vi "Visualize.vi"() -> ()   [LabVIEW 2018, in "Visualization.lvlib" / "VisualizeAcPwr.lvclass"]
uses:
  VisualizeAcPwr.lvclass
  VisualizeDigitizer/VisualizeDigitizer.lvclass
  VisualizeBase/VisualizeBase_class/Requests/clUserEventType.ctl
  <vilib>/event_ctls.llb/usereventprio.ctl
  <vilib>/Utility/error.llb/Error Cluster From Error Code.vi
  <vilib>/ErrorRing/Error Ring.xnode
  VisualizeBase/VisualizeBase_class/VisualizeBase.lvclass
  <userlib>/NIST/NISTErrorLib/NISTErrorLib.lvlib
  AcPwr/AcPwrModule/AcPwrModule.lvlib
panel:
  in  "Tab Control":enum32{"AC Instruments", "DC Instruments"}(tab)
  out "PacificPower":waveform(dbl)[](graph) caption="4140002"
  out "Chroma AC":waveform(dbl)[](graph) caption="4140003"
  out "NHRDC":waveform(sgl)[](graph) caption="-1"
  out "Chroma DC":waveform(dbl)[](graph) caption="4140003"
  out "ErrorArray":errorcluster[](array[cluster])
  in  "QueuName":string="AcPwrVisQue"
  in  "btnStop":bool
  in  "btnReset":bool
  in  "btnClear":bool
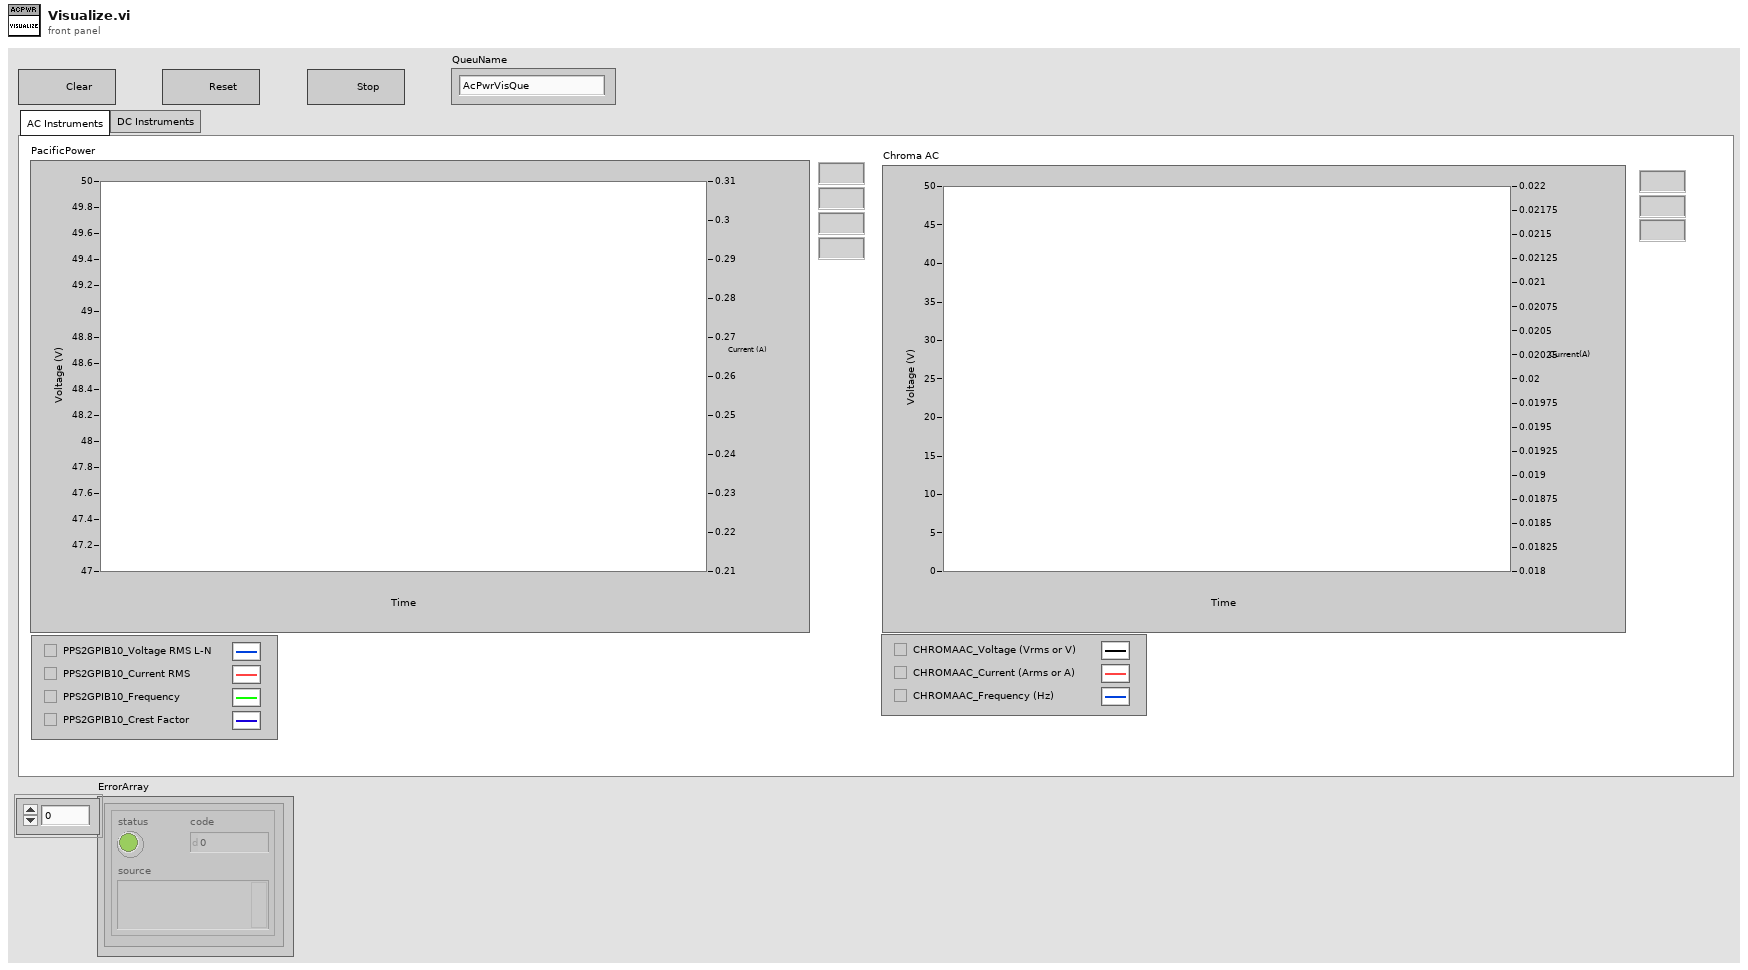
[diagram p1: front panel]
types:
  T1 = typedef "Visualization.lvlib/VisualizeBase.lvclass/clRequestEvents.ctl" = cluster{"StopRequest":refnum<user-event>, "ResetRequest":refnum<user-event>}
  T2 = typedef "AcPwrModule.lvlib/clBroadcastEvents.ctl" = cluster{"DidInit":refnum<user-event>, "StatusUpdate":refnum<user-event>, "ErrorReport":refnum<user-event>, "DidStop":refnum<user-event>, "PathToINI":refnum<user-event>, "Measurements":refnum<user-event>, "LoadConfigFile":refnum<user-event>}
  T3 = typedef "Visualization.lvlib/VisualizeBase.lvclass/clUserEventType.ctl" = cluster{"BusIndex":i8, "Data":variant}
  T4 = typedef "usereventprio.ctl" = enum32{"high priority", "normal priority"}
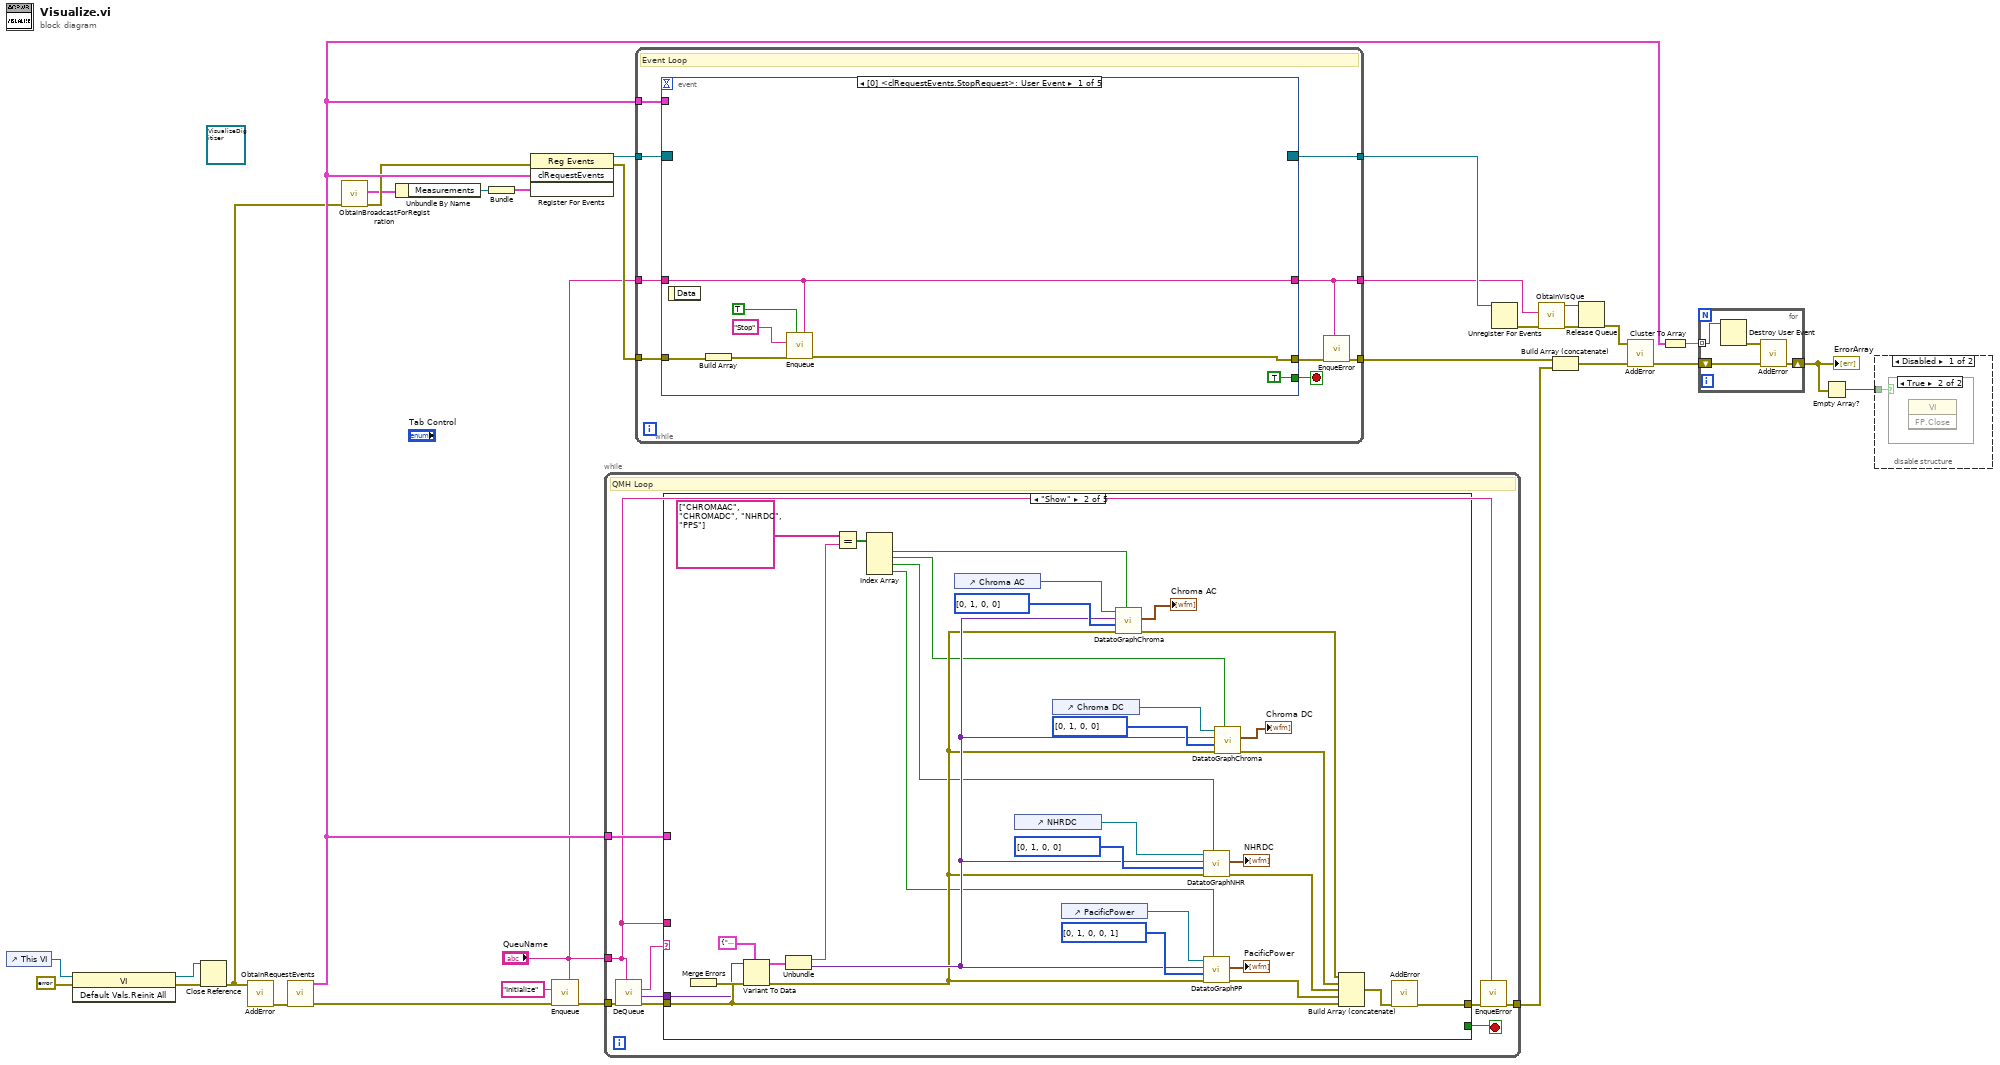
[diagram p0: block diagram]
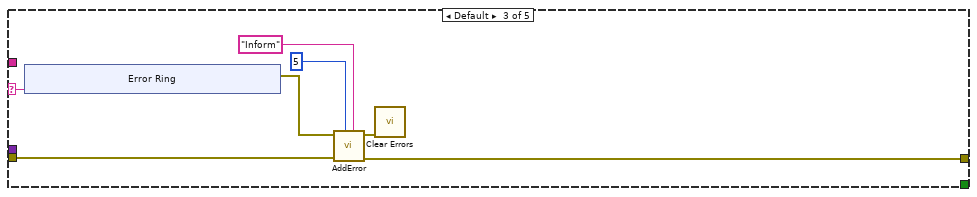
[diagram p5: hidden frame]
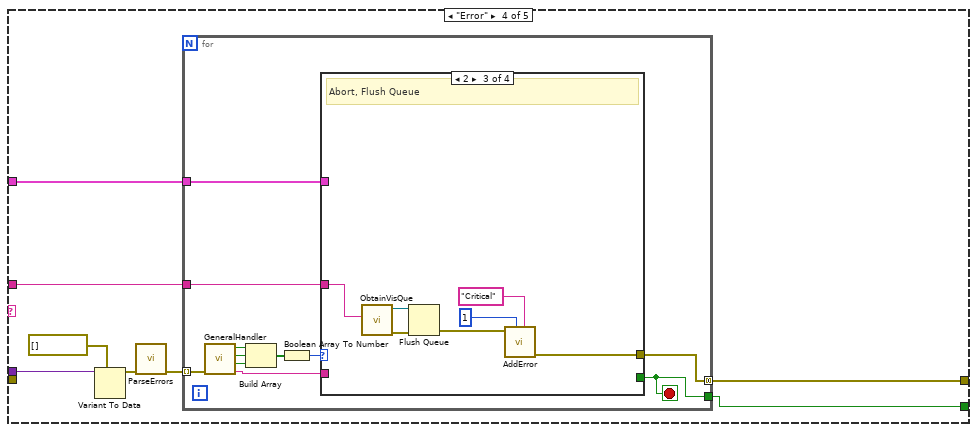
[diagram p6: hidden frame]
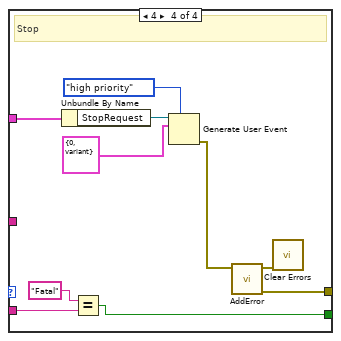
[diagram p9: hidden frame]
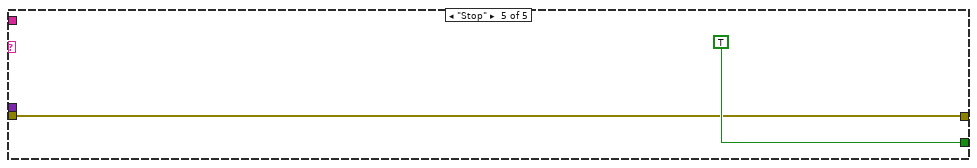
[diagram p10: hidden frame]
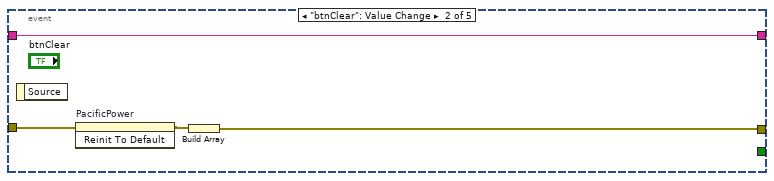
[diagram p11: hidden frame]
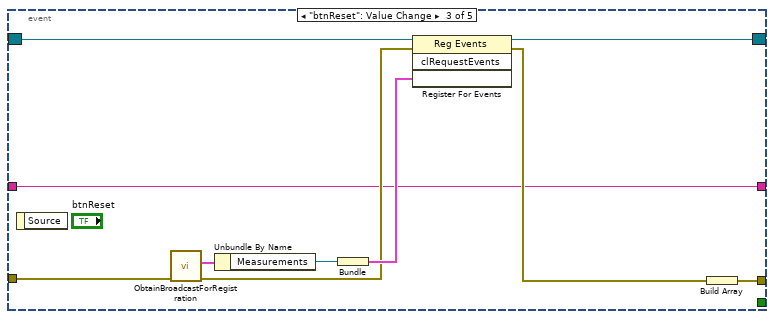
[diagram p12: hidden frame]
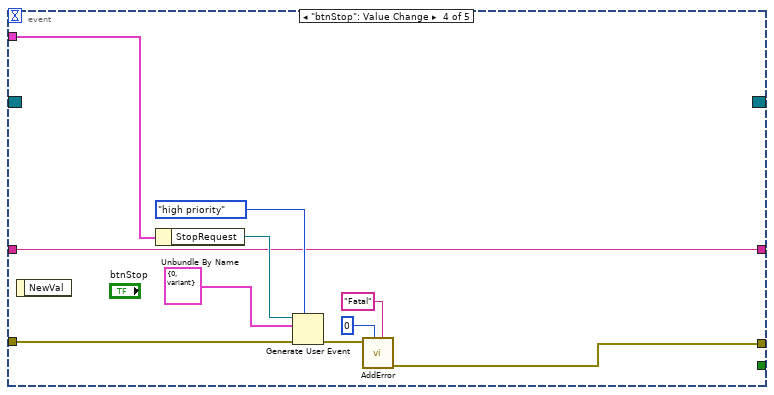
[diagram p13: hidden frame]
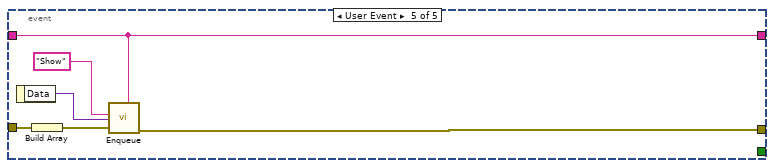
[diagram p14: hidden frame]
diagram:
  (unwired) refnum<class "VisualizeDigitizer.lvclass"> refnum ("VisualizeBase_class.lvclass")
  n1 = control-ref of="This VI"() -> (w10:refnum<vi>)
  n2 = invoke class="VI" method="Default Vals.Reinit All"(reference=w10, error in=errorcluster {"status"=FALSE, "code"=0, "source"=""} ("error in (no error)")) -> (reference out=w7:refnum<vi>, error out=w8:errorcluster)  [unwired: 1 in, 1 out]
  n3 = Close Reference(reference=w7, error in (no error)=w8) -> (error out=w5:errorcluster)
  n4 = call <userlib>:"AddError.vi"("error in (no error)"=w5) -> ("ErrorArray"=w27:errorcluster[])  [unwired: 9 in, 1 out]
  n5 = call "ObtainRequestEvents.vi"("Error"=w27) -> ("Error"=w12:errorcluster[], "clRequestEvents"=w16:T1)  [unwired: 9 in]
  n6 = call "ObtainBroadcastForRegistration.vi"("error in (no error)"=w5) -> ("error out"=w4:errorcluster, "clBroadcastEvents"=w3:T2)  [unwired: 9 in]
  n7 = Unbundle By Name(w3) -> ("Measurements"=w14:refnum<user-event>)
  n8 = Bundle("Measurements"=w14) -> (w13:cluster{"Measurements":refnum<user-event>})  [unwired: 1 in]
  n9 = register-events(error in=w4, w16, w13) -> (reference out=w28:refnum<event-registration>, error out=w11:errorcluster)  [unwired: 1 in]
  n10 = call "Enqueue.vi"("QueName"="QueuName", "Error"=w12, "Message"="Initialize") -> ("Error"=w29:errorcluster[])  [unwired: 8 in]
  n11 = while {
    tunnel: w29 -> [w39]
    tunnel: [w33] -> w23
    tunnel: "QueuName" -> [w31]
    tunnel: w16 -> [w32]
    stop <- w34 stop-if-true
    # "QMH Loop"
    n12 = call "DeQueue.vi"("QueName"=w31, "Error"=w39) -> ("Error"=w36:errorcluster[], "Data"=w37:variant, "Message"=w38:string)  [unwired: 7 in]
    n13 = case shown="\"Show\"" w38 {
      selector: w38 -> [_ _ w79 _ _]
      tunnel: w37 -> [_ w55 _ w94 _]
      tunnel: w36 -> [w40 w71 w77 _ w123]
      tunnel: [w40 w72 w76 w90 w123] -> w35
      tunnel: [_ _ _ w89 TRUE] -> w34
      tunnel: w32 -> [_ _ _ w88 _]
      tunnel: w31 -> [_ _ _ w87 _]
      frame "Initialize" {
      }
      frame "Show" {
        n14 = Merge Errors(w71) -> (w54:errorcluster)
        n15 = Variant To Data(error in=w54, type=cluster{string, "Data":variant} {"", "Data"=variant}, Variant=w55) -> (data=w56:cluster{string, "Data":variant}, error out=w46:errorcluster)
        n16 = Unbundle(w56) -> (w52:string, "Data"=w47:variant)
        n17 = Equal?(x=string[] ["CHROMAAC", "CHROMADC", "NHRDC", "PPS"], y=w52) -> (x = y?=w51:bool[])
        n18 = Index Array(array=w51) -> (element #1=w43:bool, element #2=w42:bool, element #3=w41:bool, element #4=w44:bool)  [unwired: 4 in]
        n19 = control-ref of="Chroma AC"() -> (w50:refnum<vi>)
        n20 = control-ref of="NHRDC"() -> (w63:refnum<vi>)
        n21 = control-ref of="Chroma DC"() -> (w60:refnum<vi>)
        n22 = control-ref of="PacificPower"() -> (w68:refnum<vi>)
        n23 = call "DatatoGraphChroma.vi"("Boolean"=w43, "error in (no error)"=w46, "Array 2"=u32[] [0, 1, 0, 0], "Data"=w47, "WaveformChart in"=w50) -> ("error out"=w45:errorcluster, "Array"=→"Chroma AC":waveform(dbl)[])  [unwired: 3 in, 2 out]
        n24 = call "DatatoGraphNHR.vi"("ExtractData"=w41, "error in (no error)"=w46, "Array 2"=u32[] [0, 1, 0, 0], "Data"=w47, "NHRDC WaveformChart 2"=w63) -> ("error out"=w62:errorcluster, "Array"=→"NHRDC":waveform(sgl)[])  [unwired: 4 in, 1 out]
        n25 = call "DatatoGraphPP.vi"("ExtractData"=w44, "error in (no error)"=w46, "Array 2"=u32[] [0, 1, 0, 0, 1], "Data"=w47, "PacificPowerWavefromChart 2"=w68) -> ("error out"=w66:errorcluster, "Array"=→"PacificPower":waveform(dbl)[])  [unwired: 4 in, 1 out]
        n26 = call "DatatoGraphChroma.vi"("Boolean"=w42, "error in (no error)"=w46, "Array 2"=u32[] [0, 1, 0, 0], "Data"=w47, "WaveformChart in"=w60) -> ("error out"=w58:errorcluster, "Array"=→"Chroma DC":waveform(dbl)[])  [unwired: 3 in, 2 out]
        n27 = Build Array (concatenate)(w45, w58, w62, w66, w71) -> (w70:errorcluster[])
        n28 = call <userlib>:"AddError.vi"("ErrorArray"=w70) -> ("ErrorArray"=w72:errorcluster[])  [unwired: 9 in, 1 out]
      }
      frame Default {
        n29 = xnode "Error Ring"("parameter 0"=w79) -> ("error out"=w78:errorcluster)
        n30 = call <userlib>:"AddError.vi"("Severity"="Inform" ("String"), "Priority"=u8 5, "ErrorArray"=w77, "error in (no error)"=w78) -> ("ErrorArray"=w76:errorcluster[], "error out"=w75:errorcluster)  [unwired: 6 in]
        n31 = call <vilib>:"Clear Errors.vi"("error in (no error)"=w75) -> ()  [unwired: 5 in, 2 out]
      }
      frame "Error" {
        n32 = Variant To Data(type=errorcluster[] [], Variant=w94) -> (data=w92:errorcluster[])  [unwired: 1 in, 1 out]
        n33 = call <userlib>:"ParseErrors.vi"("ErrorArray"=w92) -> ("ErrorArray"=w91:errorcluster[])  [unwired: 8 in, 2 out]
        n34 = for {
          tunnel: w91 -> [w105] mode=indexing
          tunnel: [w99] -> w90 mode=concatenating
          tunnel: [w97] -> w89
          tunnel: w88 -> [w96]
          tunnel: w87 -> [w95]
          stop <- w97 stop-if-true
          n35 = call <userlib>:"GeneralHandler.vi"("error in (no error)"=w105) -> ("Severity"=w98:string, "Stop"=w102:bool, "Abort"=w103:bool, "Continue"=w104:bool)  [unwired: 7 in]
          n36 = Build Array(w104, w103, w102) -> (w101:bool[])
          n37 = Boolean Array To Number(Boolean array=w101) -> (number=w100:u32)
          n38 = case shown="2" w100 {
            tunnel: [_ _ w110 w121] -> w99
            tunnel: w98 -> [_ _ _ w116]
            tunnel: [_ _ _ w114] -> w97
            tunnel: w96 -> [_ _ _ w113]
            tunnel: w95 -> [_ _ w106 _]
            frame 0, Default {
              # "No Dialog"
            }
            frame 1 {
              # "Continue"
            }
            frame 2 {
              # "Abort, Flush Queue"
              n39 = call "ObtainVisQue.vi"("QueName"=w106) -> ("error out"=w112:errorcluster, "queue out"=w111:refnum<queue>)  [unwired: 9 in]
              n40 = Flush Queue(queue=w111, error in (no error)=w112) -> (error out=w109:errorcluster)  [unwired: 2 out]
              n41 = call <userlib>:"AddError.vi"("Severity"="Critical" ("String"), "Priority"=u8 1, "error in (no error)"=w109) -> ("ErrorArray"=w110:errorcluster[])  [unwired: 7 in, 1 out]
            }
            frame 4 {
              # "Stop"
              n42 = Unbundle By Name(w113) -> ("StopRequest"=w122:refnum<user-event>)
              n43 = Equal?(x="Fatal", y=w116) -> (x = y?=w114:bool)
              n44 = Generate User Event(priority (normal)=usereventprio."high priority", user event=w122, event data cluster=T3 {"BusIndex"=0, "Data"=variant} ("event data")) -> (error out=w120:errorcluster)  [unwired: 1 in, 1 out]
              n45 = call <userlib>:"AddError.vi"("error in (no error)"=w120) -> ("ErrorArray"=w121:errorcluster[], "error out"=w117:errorcluster)  [unwired: 9 in]
              n46 = call <vilib>:"Clear Errors.vi"("error in (no error)"=w117) -> ()  [unwired: 5 in, 2 out]
            }
          }
        }
      }
      frame "Stop" {
      }
    }
    n47 = call "EnqueError.vi"("QueName"=w31, "Error"=w35) -> ("Error"=w33:errorcluster[])  [unwired: 9 in]
  }
  n48 = while {
    tunnel: w28 -> [w133]
    tunnel: [w130] -> w24
    tunnel: [w129] -> w26
    tunnel: w16 -> [w128]
    tunnel: w11 -> [w127]
    tunnel: "QueuName" -> [w126]
    tunnel: [w125] -> w1
    stop <- w132 stop-if-true
    # "Event Loop"
    n49 = event shown="[0] <clRequestEvents.StopRequest>: User Event" {
      selector: w133 -> [_ _ w154 _ _]
      dyn-events: [_ _ w153 _ _] -> w129
      timeout: _ -> [_ _ _ _ _]
      tunnel: [TRUE _ _ _ _] -> w132
      tunnel: [w139 w144 w148 w162 w168] -> w131
      tunnel: w128 -> [_ _ _ w157 _]
      tunnel: w127 -> [w136 w143 w150 w156 w166]
      tunnel: w126 -> [w134 w141 w145 w155 w167]
      tunnel: [w134 w141 w145 w155 w167] -> w125
      event User Event {
        n50 = event-data() -> ()  [unwired: 1 in, 1 out]
        n51 = Build Array(w136) -> (w135:errorcluster[])
        n52 = call "Enqueue.vi"("QueName"=w134, "Priority? (F)"=TRUE, "Error"=w135, "Message"="Stop") -> ("Error"=w139:errorcluster[])  [unwired: 7 in]
      }
      event "btnClear": Value Change {
        n53 = event-data() -> ()  [unwired: 1 in, 1 out]
        n54 = invoke on="PacificPower" class="WFChart (strict)" method="Reinit To Default"(error in=w143) -> (error out=w142:errorcluster)  [unwired: 2 in, 2 out]
        n55 = Build Array(w142) -> (w144:errorcluster[])
      }
      event "btnReset": Value Change {
        n56 = event-data() -> ()  [unwired: 1 in, 1 out]
        n57 = call "ObtainBroadcastForRegistration.vi"("error in (no error)"=w150) -> ("error out"=w147:errorcluster, "clBroadcastEvents"=w149:T2)  [unwired: 9 in]
        n58 = Unbundle By Name(w149) -> ("Measurements"=w152:refnum<user-event>)
        n59 = Bundle("Measurements"=w152) -> (w151:cluster{"Measurements":refnum<user-event>})  [unwired: 1 in]
        n60 = register-events(reference=w154, error in=w147, w151) -> (reference out=w153:refnum<event-registration>, error out=w146:errorcluster)  [unwired: 1 in]
        n61 = Build Array(w146) -> (w148:errorcluster[])
      }
      event "btnStop": Value Change {
        n62 = event-data() -> ()  [unwired: 1 in, 1 out]
        n63 = Unbundle By Name(w157) -> ("StopRequest"=w163:refnum<user-event>)
        n64 = Generate User Event(priority (normal)=usereventprio."high priority", user event=w163, event data cluster=T3 {"BusIndex"=0, "Data"=variant} ("event data"), error in=w156) -> (error out=w164:errorcluster)  [unwired: 1 out]
        n65 = call <userlib>:"AddError.vi"("Severity"="Fatal" ("String"), "Priority"=u8 0, "error in (no error)"=w164) -> ("ErrorArray"=w162:errorcluster[])  [unwired: 7 in, 1 out]
      }
      event User Event {
        n66 = event-data() -> ("Data"=w170:variant)  [unwired: 1 in]
        n67 = Build Array(w166) -> (w165:errorcluster[])
        n68 = call "Enqueue.vi"("QueName"=w167, "Error"=w165, "Data"=w170, "Message"="Show") -> ("Error"=w168:errorcluster[])  [unwired: 7 in]
      }
    }
    n69 = call "EnqueError.vi"("QueName"=w125, "Error"=w131) -> ("Error"=w130:errorcluster[])  [unwired: 9 in]
  }
  n70 = Unregister For Events(event registration refnum=w26) -> (error out=w22:errorcluster)  [unwired: 1 in]
  n71 = call "ObtainVisQue.vi"("error in (no error)"=w22, "QueName"=w1) -> ("error out"=w20:errorcluster, "queue out"=w19:refnum<queue>)  [unwired: 8 in]
  n72 = Build Array (concatenate)(w24, w23) -> (w21:errorcluster[])
  n73 = Release Queue(queue=w19, error in (no error)=w20) -> (error out=w18:errorcluster)  [unwired: 1 in, 2 out]
  n74 = call <userlib>:"AddError.vi"("ErrorArray"=w21, "error in (no error)"=w18) -> ("ErrorArray"=w17:errorcluster[])  [unwired: 8 in, 1 out]
  n75 = Cluster To Array(cluster=w16) -> (array=w25:refnum<user-event>[])
  n76 = for {
    tunnel: w25 -> [w174] mode=indexing
    shift-right: [w173] -> w6
    shift-left: w17 -> [w172]
    n77 = Destroy User Event(user event=w174) -> (error out=w171:errorcluster)  [unwired: 1 in]
    n78 = call <userlib>:"AddError.vi"("ErrorArray"=w172, "error in (no error)"=w171) -> ("ErrorArray"=w173:errorcluster[])  [unwired: 8 in, 1 out]
  }
  "ErrorArray" <- w6
  n79 = Empty Array?(array=w6) -> (empty?=w15:bool)
  n80 = disable-structure shown="Disabled" {
    disable-tunnel: w15 -> [w175 _]
    frame Disabled {
      n81 = case shown="True" w175 {
        frame False {
        }
        frame True {
          n82 = invoke class="VI" method="FP.Close"() -> ()  [unwired: 3 in, 3 out]
        }
      }
    }
    frame Enabled {
    }
  }
